vi "NT Format Generic  to Config String.vi"(11 "Field Value":T1) -> (3 "String":string)   [LabVIEW 2017]
doc: "Format the generic union data into a string."
uses:
  <vilib>/Rock Robotics/Network Tables/Field Data.ctl
  <vilib>/Rock Robotics/Network Tables/Field Type.ctl
  <vilib>/Rock Robotics/Network Tables/Sequence.ctl
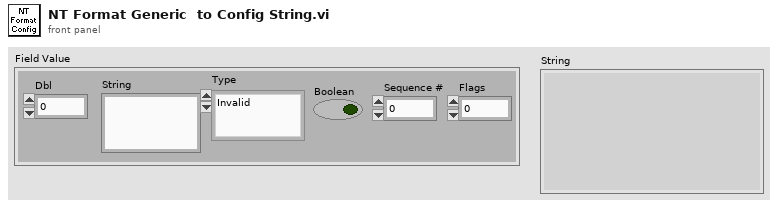
[diagram p1: front panel]
types:
  T1 = typedef "Field Data.ctl" = cluster{"Dbl":dbl, "String":string, "Type":T2, "Boolean":bool, "Sequence #":T3, "Flags":u8}
  T2 = typedef "Field Type.ctl" = enum8{"Invalid", "Bool", "Numeric", "String", "Raw", "Boolean Array", "Numeric Array", "String Array", "RPC"}
  T3 = typedef "Sequence.ctl" = u16
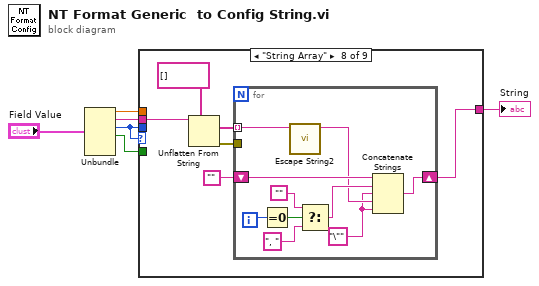
[diagram p0: block diagram]
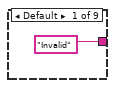
[diagram p2: hidden frame]
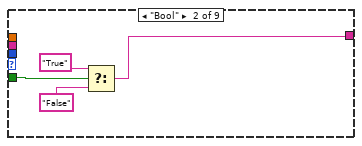
[diagram p3: hidden frame]
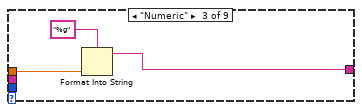
[diagram p4: hidden frame]
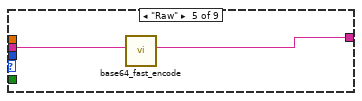
[diagram p6: hidden frame]
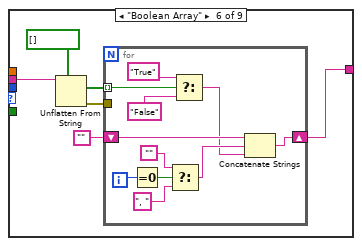
[diagram p7: hidden frame]
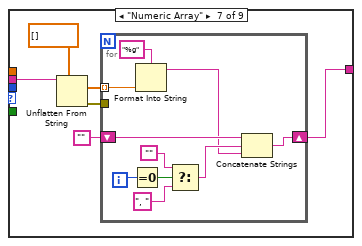
[diagram p8: hidden frame]
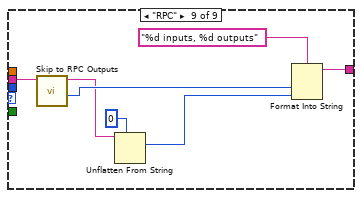
[diagram p9: hidden frame]
diagram:
  n1 = Unbundle("Field Value") -> ("Dbl"=w5:dbl, "String"=w4:string, "Type"=w2:T2, "Boolean"=w1:bool)  [unwired: 2 out]
  n2 = case shown="\"String Array\"" w2 {
    tunnel: w1 -> [_ w9 _ _ _ _ _ _ _]
    tunnel: w2 -> [_ _ _ _ _ _ _ _ _]
    tunnel: w4 -> [_ _ _ w15 w17 w22 w40 w56 w71]
    tunnel: w5 -> [_ _ w14 _ _ _ _ _ _]
    tunnel: ["Invalid" w8 w13 w15 w16 w19 w37 w53 w73] -> w6
    frame Default {
    }
    frame "Bool" {
      n3 = Select(t="True", s=w9, f="False") -> (s? t:f=w8:string)
    }
    frame "Numeric" {
      n4 = Format Into String(format string="%g", w14) -> (resulting string=w13:string)  [unwired: 2 in, 1 out]
    }
    frame "String" {
    }
    frame "Raw" {
      n5 = call <vilib>:"base64_fast_encode.vi"("string in (not encoded)"=w17) -> ("string out (base64-encoded)"=w16:string)  [unwired: 9 in, 1 out]
    }
    frame "Boolean Array" {
      n6 = Unflatten From String(type=bool[] [], binary string=w22) -> (value=w21:bool[], error out=w18:errorcluster)  [unwired: 3 in, 1 out]
      n7 = for {
        tunnel: w21 -> [w32] mode=indexing
        shift-right: [w25] -> w19
        shift-left: "" -> [w31]
        tunnel: w18 -> [_]
        i -> [w30]
        n8 = Equal To 0?(x=w30) -> (x = 0?=w29:bool)
        n9 = Select(t="", s=w29, f=", ") -> (s? t:f=w26:string)
        n10 = Select(t="True", s=w32, f="False") -> (s? t:f=w24:string)
        n11 = Concatenate Strings(w31, w26, w24) -> (w25:string)
      }
    }
    frame "Numeric Array" {
      n12 = Unflatten From String(type=dbl[] [], binary string=w40) -> (value=w39:dbl[], error out=w35:errorcluster)  [unwired: 3 in, 1 out]
      n13 = for {
        tunnel: w39 -> [w43] mode=indexing
        shift-right: [w44] -> w37
        shift-left: "" -> [w50]
        tunnel: w35 -> [_]
        i -> [w49]
        n14 = Equal To 0?(x=w49) -> (x = 0?=w48:bool)
        n15 = Format Into String(format string="%g", w43) -> (resulting string=w41:string)  [unwired: 2 in, 1 out]
        n16 = Select(t="", s=w48, f=", ") -> (s? t:f=w45:string)
        n17 = Concatenate Strings(w50, w45, w41) -> (w44:string)
      }
    }
    frame "String Array" {
      n18 = Unflatten From String(type=string[] [], binary string=w56) -> (value=w55:string[], error out=w51:errorcluster)  [unwired: 3 in, 1 out]
      n19 = for {
        tunnel: w55 -> [w59] mode=indexing
        shift-right: [w60] -> w53
        shift-left: "" -> [w66]
        tunnel: w51 -> [_]
        i -> [w65]
        w57 = "\""
        n20 = Equal To 0?(x=w65) -> (x = 0?=w64:bool)
        n21 = call <vilib>:"Escape String2.vi"("input"=w59) -> ("output"=w58:string)  [unwired: 10 in]
        n22 = Select(t="", s=w64, f=", ") -> (s? t:f=w61:string)
        n23 = Concatenate Strings(w66, w61, w57, w58, w57) -> (w60:string)
      }
    }
    frame "RPC" {
      n24 = call <vilib>:"Skip to RPC Outputs.vi"("String in"=w71) -> ("inputs"=w70:u8, "String out"=w68:string)  [unwired: 8 in, 1 out]
      n25 = Unflatten From String(type=u8 0 ("bytes to read"), binary string=w68) -> (value=w67:u8)  [unwired: 3 in, 2 out]
      n26 = Format Into String(format string="%d inputs, %d outputs", w70, w67) -> (resulting string=w73:string)  [unwired: 2 in, 1 out]
    }
  }
  "String" <- w6
